vi "initialize.vi"(0 "HGF_SVEvent":refnum<class "HGF_SVEvent.lvclass">, 3 "initializationData":variant, 5 "error in (no error)":errorcluster, 7 "binaryString":string, 8 "I8 Array":i8[](array[numeric]), 9 "prependSize? (T)":bool, 11 "byteOrder (0:big-endian, network order)":T1(ring)) -> (14 "dup HGF_SVEvent":refnum<class "HGF_SVEvent.lvclass">, 17 "found?":bool, 19 "error out":errorcluster)   [LabVIEW 2012, in "HGF_SV.lvlib" / "HGF_SVEvent.lvclass"]
doc: "This is a dynamic dispatch VI to be implemented by child classes to initialize their attributes.\n\n<B>Recommendation:</B> Use Variant for initialization data."
uses:
  HGF_SVEvent.lvclass
  HGF_BaseClasses/HGF_NetworkVisitor/HGF_NetworkVisitor.lvclass
  HGF_BaseClasses/HGF_TriggeredEvent/HGF_TriggeredEvent.lvclass
  HGF_BaseClasses/HGF_NetworkEvent/HGF_NetworkEvent.lvclass/HGF_NetworkEvent.lvclass
  HGF_SVEvent.lvclass/HGF_SVEvent.ctl
  HGF_SVCommand/HGF_SVCommand.lvclass
  HGF_SVFactory/HGF_SVFactory.lvclass
  HGF_SVSubscriber/HGF_SVSubscriber.lvclass
  HGF_BaseClasses/HGF_Factory/HGF_Factory.lvclass
  Visitors/HGF_SVMonitorVisitor_register/HGF_SVMonitorVisitor_register.lvclass
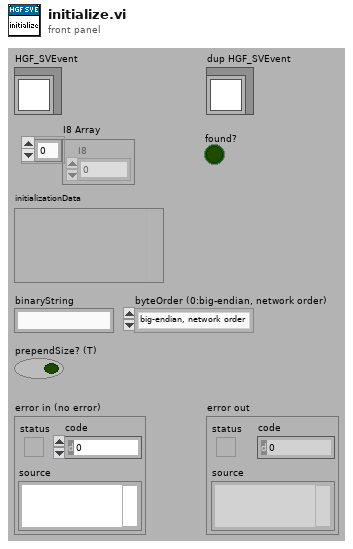
[diagram p1: front panel]
types:
  T1 = enum16{"big-endian, network order", "native, host order", "little-endian"}
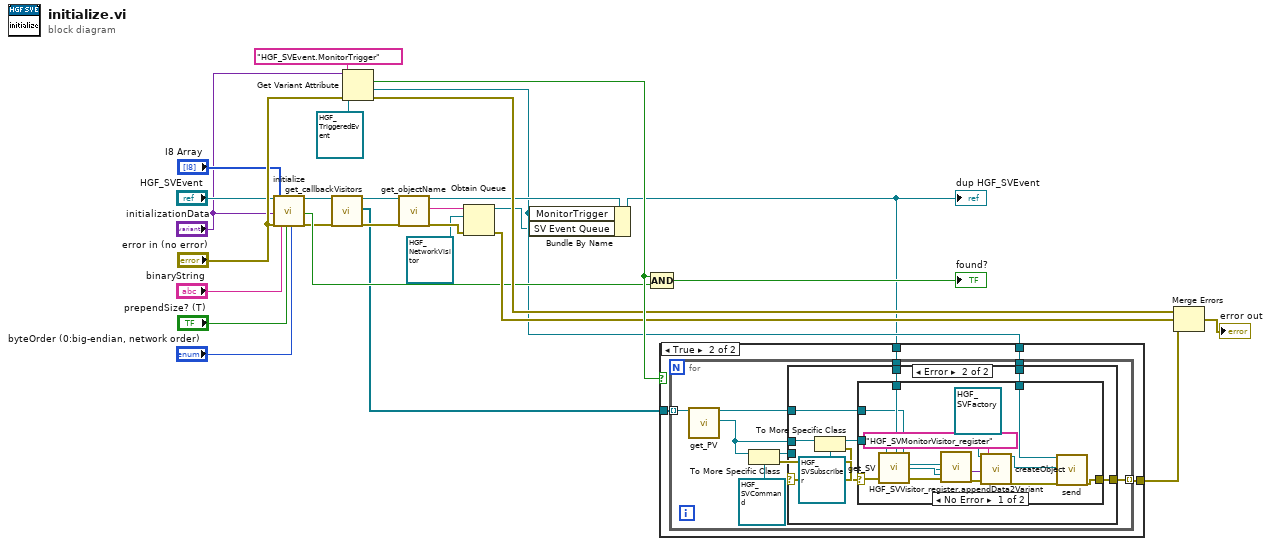
[diagram p0: block diagram]
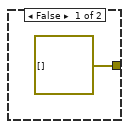
[diagram p2: hidden frame]
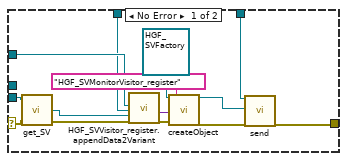
[diagram p3: hidden frame]
diagram:
  n1 = call-parent "initialize.vi"("HGF_NetworkEvent"="HGF_SVEvent", "initializationData"="initializationData", "error in (no error)"="error in (no error)", "binaryString"="binaryString", "I8 Array"="I8 Array", "prependSize? (T)"="prependSize? (T)", "byteOrder (0:big-endian, network order)"="byteOrder (0:big-endian, network order)") -> ("dup HGF_NetworkEvent"=w14:refnum<class "HGF_SVEvent.lvclass">, "found?"=w17:bool, "error out"=w15:errorcluster)  [unwired: 10 out]
  n2 = call "get_callbackVisitors.vi"("HGF_NetworkEvent"=w14, "error in (no error)"=w15) -> ("dup HGF_NetworkEvent"=w8:refnum<class "HGF_SVEvent.lvclass">, "callbackVisitors"=w7:refnum<class "HGF_NetworkVisitor.lvclass">[], "error out"=w13:errorcluster)  [unwired: 15 out]
  n3 = Get Variant Attribute(Variant="initializationData", name="HGF_SVEvent.MonitorTrigger", default value (empty Variant)=refnum<class "HGF_TriggeredEvent.lvclass"> refnum ("HGF_BaseClasses.lvlib:HGF_TriggeredEvent.lvclass"), error in="error in (no error)") -> (found=w28:bool, value=w6:refnum<class "HGF_TriggeredEvent.lvclass">, error out=w26:errorcluster)  [unwired: 1 out]
  n4 = call "get_objectName.vi"("HGF_Factory"=w8, "error in (no error)"=w13) -> ("dup HGF_Factory"=w12:refnum<class "HGF_SVEvent.lvclass">, "objectName"=w9:string, "error out"=w11:errorcluster)  [unwired: 15 out]
  n5 = Obtain Queue(name (unnamed)=w9, element data type=refnum<class "HGF_NetworkVisitor.lvclass"> refnum ("HGF_BaseClasses.lvlib:HGF_NetworkVisitor.lvclass"), error in (no error)=w11) -> (queue out=w5:refnum<queue>, error out=w27:errorcluster)  [unwired: 2 in, 1 out]
  n6 = Bundle By Name(cluster=w12, "MonitorTrigger"=w6, "SV Event Queue"=w5) -> (w1:refnum<class "HGF_SVEvent.lvclass">)
  "dup HGF_SVEvent" <- w1
  n7 = Compound Arithmetic op=AND(w28, w17) -> (→"found?":bool)
  n8 = case shown="True" w28 {
    tunnel: w7 -> [_ w33]
    tunnel: w6 -> [_ w32]
    tunnel: [errorcluster[] [] w31] -> w4
    tunnel: w1 -> [_ w30]
    frame False {
    }
    frame True {
      n9 = for {
        tunnel: w33 -> [w42] mode=indexing
        tunnel: w32 -> [w37]
        tunnel: [w35] -> w31 mode=indexing
        tunnel: w30 -> [w34]
        n10 = call "get_PV.vi"("HGF_NetworkData"=w42) -> ("dup HGF_NetworkData"=w36:refnum<class "HGF_NetworkVisitor.lvclass">, "HGV_PVBase"=w39:refnum<class "HGF_PVBase.lvclass">)  [unwired: 1 in, 16 out]
        n11 = To More Specific Class(target class=refnum<class "HGF_SVCommand.lvclass"> refnum ("HGF_SV.lvlib:HGF_SVCommand.lvclass"), reference=w39) -> (specific class reference=w38:refnum<class "HGF_SVCommand.lvclass">, error out=w40:errorcluster)  [unwired: 1 in]
        n12 = case shown="Error" w40 {
          selector: w40 -> [w56 _]
          tunnel: w39 -> [_ w64]
          tunnel: w38 -> [w55 _]
          tunnel: w37 -> [w47 w57]
          tunnel: w36 -> [w50 w60]
          tunnel: [w46 w59] -> w35
          tunnel: w34 -> [w49 w58]
          frame No Error {
            n13 = call-dynamic "get_SV.vi"("error in (no error)"=w56, "HGF_SVCommand"=w55) -> ("error out"=w48:errorcluster, "shared variable refnum"=w43:refnum<k21>)  [unwired: 1 in, 1 out]
            n14 = call "HGF_SVVisitor_register.appendData2Variant.vi"("HGF_NetworkVisitor"=w50, "HGF_TriggeredEvent"=w49, "shared variable refnum (without DSC)"=w43, "error in"=w48) -> ("dup variant"=w52:variant, "error out"=w51:errorcluster)  [unwired: 14 in]
            n15 = call "createObject.vi"("HGF_Factory"=refnum<class "HGF_SVFactory.lvclass"> refnum ("HGF_SV.lvlib:HGF_SVFactory.lvclass"), "initializationData"=w52, "error in (no error)"=w51, "className"="HGF_SVMonitorVisitor_register") -> ("HGF_Object"=w45:refnum<class "HGF_Factory.lvclass">, "error out"=w44:errorcluster)  [unwired: 13 in, 1 out]
            n16 = call-dynamic "send.vi"("HGF_Event"=w47, "Object"=w45, "error in (no error)"=w44) -> ("error out"=w46:errorcluster)  [unwired: 14 in, 2 out]
          }
          frame Error {
            n17 = To More Specific Class(target class=refnum<class "HGF_SVSubscriber.lvclass"> refnum ("HGF_SV.lvlib:HGF_SVSubscriber.lvclass"), reference=w64) -> (specific class reference=w61:refnum<class "HGF_SVSubscriber.lvclass">, error out=w62:errorcluster)  [unwired: 1 in]
            n18 = case shown="No Error" w62 {
              selector: w62 -> [w77 w79]
              tunnel: w61 -> [w78 _]
              tunnel: w60 -> [w67 _]
              tunnel: [w65 w79] -> w59
              tunnel: w58 -> [w68 _]
              tunnel: w57 -> [w66 _]
              frame No Error {
                n19 = call-dynamic "get_SV.vi"("error in (no error)"=w77, "HGF_SVSubscriber"=w78) -> ("error out"=w70:errorcluster, "shared variable refnum"=w69:refnum<k21>)  [unwired: 1 in, 1 out]
                n20 = call "HGF_SVVisitor_register.appendData2Variant.vi"("HGF_NetworkVisitor"=w67, "HGF_TriggeredEvent"=w68, "shared variable refnum (without DSC)"=w69, "error in"=w70) -> ("dup variant"=w74:variant, "error out"=w73:errorcluster)  [unwired: 14 in]
                n21 = call "createObject.vi"("HGF_Factory"=refnum<class "HGF_SVFactory.lvclass"> refnum ("HGF_SV.lvlib:HGF_SVFactory.lvclass"), "initializationData"=w74, "error in (no error)"=w73, "className"="HGF_SVMonitorVisitor_register") -> ("HGF_Object"=w72:refnum<class "HGF_Factory.lvclass">, "error out"=w71:errorcluster)  [unwired: 13 in, 1 out]
                n22 = call-dynamic "send.vi"("HGF_Event"=w66, "Object"=w72, "error in (no error)"=w71) -> ("error out"=w65:errorcluster)  [unwired: 14 in, 2 out]
              }
              frame Error {
              }
            }
          }
        }
      }
    }
  }
  n23 = Merge Errors(w26, w27, w4) -> (→"error out":errorcluster)
